vi "Prompt for Step.vi"(8 "error in (no error)":errorcluster, 10 "Subpanel Ref":refnum<vi>, 11 "Boolean Assertion in":refnum<class "Boolean Assertion.lvclass">) -> (0 "error out":errorcluster, 3 "Boolean Assertion out":refnum<class "Boolean Assertion.lvclass">)   [LabVIEW 2020, in "MacroAssert.lvlib" / "Boolean Assertion.lvclass"]
doc: "Displays its own window into <B>Subpanel Ref</B> for the user to enter a macro step."
uses:
  Boolean Assertion.lvclass
  Assertion Step/Assertion Step.lvclass
panel:
  in  "Object Name":string
  in  "Comparison Value":bool
  out "Subtype Description":string
  in  "Step Subtype":u16(ring) items=["Boolean Ctl Value", "Ctl Visible Property", "Ctl is Enabled", "Ctl is Grayed Out", "Ctl Key Focus Property", "VI Front Panel is Open", "Window is in Running Windows", "Window is in Monitor Bounds"]
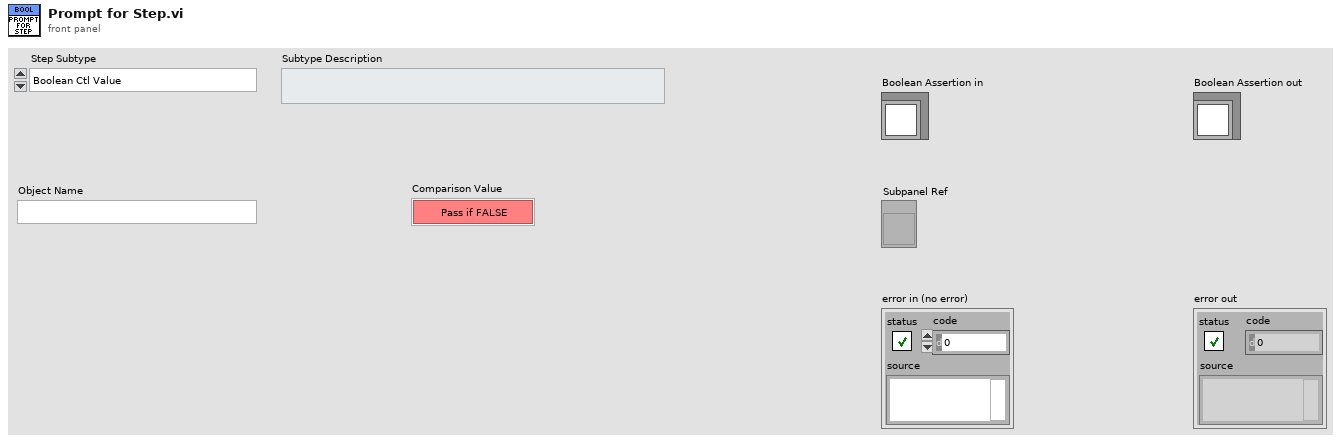
[diagram p1: front panel]
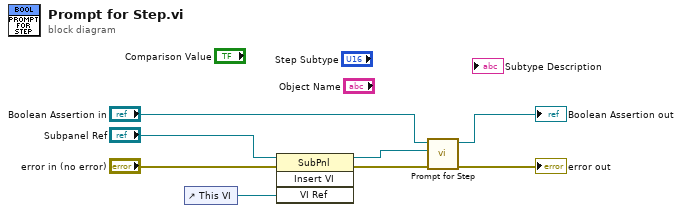
[diagram p0: block diagram]
diagram:
  n1 = control-ref of="This VI"() -> (w6:refnum<vi>)
  n2 = invoke class="SubPnl" method="Insert VI"(reference="Subpanel Ref", error in="error in (no error)", "VI Ref"=w6) -> (reference out=w7:refnum<vi>, error out=w8:errorcluster)  [unwired: 1 in, 2 out]
  n3 = call-parent "Prompt for Step.vi"("error in (no error)"=w8, "Subpanel Ref"=w7, "Step in"="Boolean Assertion in") -> ("error out"=→"error out":errorcluster, "Step out"=→"Boolean Assertion out":refnum<class "Boolean Assertion.lvclass">)  [unwired: 7 in]
